vi "number-to-match.vi"() -> ()   [LabVIEW 2023]
panel:
  in  "?":bool
  out "Iteration Count":i32
  in  "Number to Match":dbl
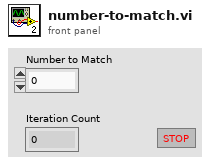
[diagram p1: front panel]
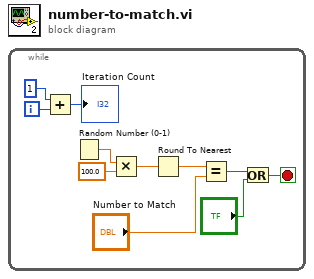
[diagram p0: block diagram]
diagram:
  n1 = while {
    i -> [w1]
    stop <- w5 stop-if-true
    n2 = Add(x=1, y=w1) -> (x+y=→"Iteration Count":i32)
    n3 = Random Number (0-1)() -> (number: 0 to 1=w11:dbl)
    n4 = Multiply(x=w11, y=100.0) -> (x*y=w9:dbl)
    n5 = Round To Nearest(number=w9) -> (nearest integer value=w4:dbl)
    n6 = Equal?(x=w4, y="Number to Match") -> (x = y?=w7:bool)
    n7 = Or(x=w7, y="?") -> (x .or. y?=w5:bool)
  }
